vi "Table Function - Cut to Ext-Clipboard.vi"(8 "error in":errorcluster, 9 "Selection Size":T1, 10 "Selection Start":T1, 11 "Text Table":string[][](array[string])) -> (0 "error out":errorcluster, 1 "Cut Section to Clipboard":string[][](array[string]), 3 "Table minus Cut Section":string[][](array[string]))   [LabVIEW 2018]
uses:
  <vilib>/Utility/miscctls.llb/LVRowAndColumnTypeDef.ctl
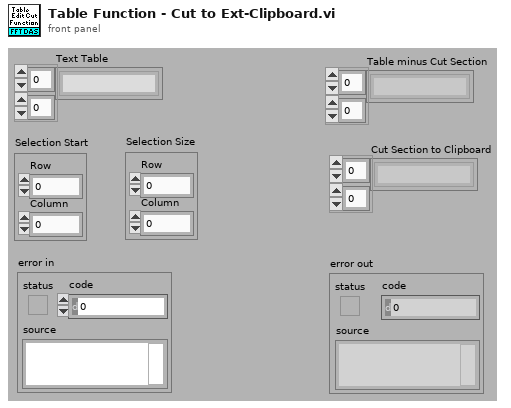
[diagram p1: front panel]
types:
  T1 = typedef "LVRowAndColumnTypeDef.ctl" = cluster{"Row":i32, "Column":i32}
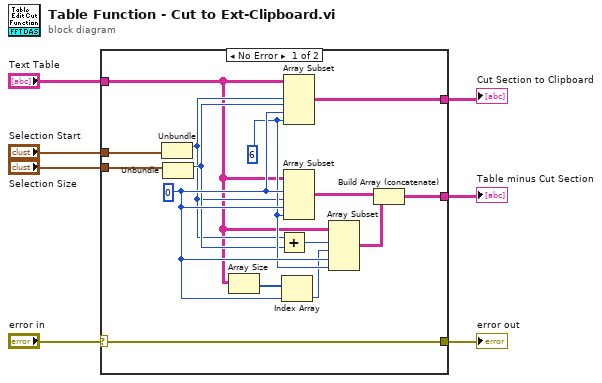
[diagram p0: block diagram]
diagram:
  n1 = case shown="No Error" "error in" {
    selector: "error in" -> [w8 w23]
    tunnel: "Selection Size" -> [w22 _]
    tunnel: "Selection Start" -> [w21 _]
    tunnel: [w14 w24] -> w5
    tunnel: "Text Table" -> [w13 w24]
    tunnel: [w9 _] -> w3
    tunnel: [w8 w23] -> w1
    frame No Error {
      w19 = 6
      w20 = 0
      n2 = Unbundle(w21) -> ("Row"=w15:i32)  [unwired: 1 out]
      n3 = Unbundle(w22) -> ("Row"=w16:i32)  [unwired: 1 out]
      n4 = Array Size(array=w13) -> (size(s)=w12:i32[])
      n5 = Add(x=w15, y=w16) -> (x+y=w10:i32)
      n6 = Index Array(array=w12, index=w20) -> (element=w11:i32)
      n7 = Array Subset(array=w13, index (row)=w15, length (row)=w16, index (col)=w20, length (col)=w19) -> (w9:string[][])
      n8 = Array Subset(array=w13, index (row)=w20, length (row)=w15, index (col)=w20, length (col)=w19) -> (w17:string[][])
      n9 = Array Subset(array=w13, index (row)=w10, length (row)=w11, index (col)=w20, length (col)=w19) -> (w18:string[][])
      n10 = Build Array (concatenate)(w17, w18) -> (w14:string[][])
    }
    frame Error {
    }
  }
  "Table minus Cut Section" <- w5
  "Cut Section to Clipboard" <- w3
  "error out" <- w1
